vi "Create range template.vi"(8 "error in":errorcluster, 9 "Range Template (А..Я)":string="А..Я") -> (0 "error out":errorcluster, 1 "first Letter":string, 2 "last Letter":string, 3 "Template String":string)   [LabVIEW 2018]
doc: "Формирование алфавита для построения команд протокола обмена с подсистемами АСНИ и АСУ"
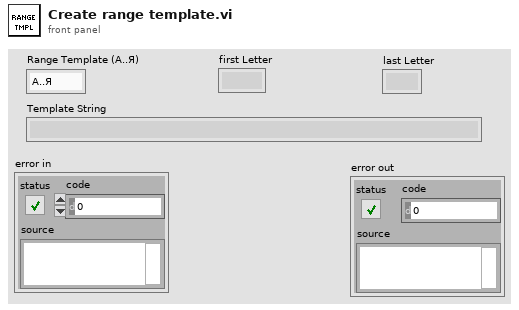
[diagram p1: front panel]
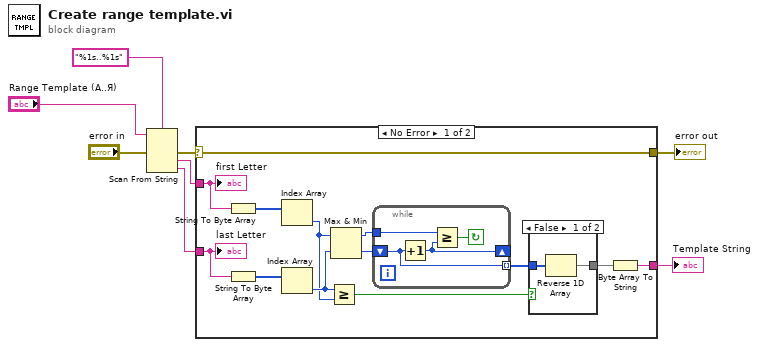
[diagram p0: block diagram]
diagram:
  n1 = Scan From String(format string="%1s..%1s", input string="Range Template (А..Я)", error in="error in") -> (error out=w2:errorcluster, output 1=w5:string, output 2=w4:string)  [unwired: 3 in, 2 out]
  n2 = case shown="No Error" w2 {
    selector: w2 -> [w16 w29]
    tunnel: w5 -> [w21 _]
    tunnel: w4 -> [w19 _]
    tunnel: [w17 _] -> w3
    tunnel: [w16 w29] -> w1
    frame No Error {
      n3 = String To Byte Array(string=w21) -> (unsigned byte array=w20:u8[])
      n4 = String To Byte Array(string=w19) -> (unsigned byte array=w18:u8[])
      n5 = Index Array(array=w20) -> (element=w12:u8)  [unwired: 1 in]
      n6 = Index Array(array=w18) -> (element=w13:u8)  [unwired: 1 in]
      n7 = Greater Or Equal?(x=w13, y=w12) -> (x >= y?=w9:bool)
      n8 = Max & Min(x=w12, y=w13) -> (max(x,y)=w15:u8, min(x,y)=w14:u8)
      n9 = while {
        tunnel: [w27] -> w10 mode=indexing
        tunnel: w15 -> [w26]
        shift-right: [w25] -> _
        shift-left: w14 -> [w27]
        stop <- w28 continue-if-true
        n10 = Increment(x=w27) -> (x+1=w25:u8)
        n11 = Greater Or Equal?(x=w26, y=w25) -> (x >= y?=w28:bool)
      }
      n12 = case shown="False" w9 {
        tunnel: [w22 w24] -> w11
        tunnel: w10 -> [w23 w24]
        frame False {
          n13 = Reverse 1D Array(array=w23) -> (reversed array=w22:u8[])
        }
        frame True {
        }
      }
      n14 = Byte Array To String(unsigned byte array=w11) -> (string=w17:string)
      "first Letter" <- w21
      "last Letter" <- w19
    }
    frame Error {
    }
  }
  "error out" <- w1
  "Template String" <- w3
